vi "testRotGroupDOF.vi"(8 "error in (no error)":errorcluster) -> (0 "error out":errorcluster)   [LabVIEW 2016]
doc: "Test the rotation of degree of freedom (DOF) with the non-zero camera rotation angle."
uses:
  CamRot/CamRot.lvclass
  StrictDef/DofGroup.ctl
  <vilib>/addons/_JKI Toolkits/Caraya/classes/Test/Test.lvclass
  <vilib>/addons/_JKI Toolkits/Caraya/classes/Assert/Assert.lvclass
panel:
  in  "CamRot.lvclass":refnum<class "CamRot.lvclass">
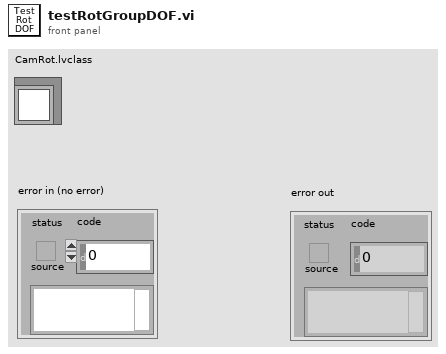
[diagram p1: front panel]
types:
  T1 = typedef "DofGroup.ctl" = enum16{"M2 Hex Pos", "Cam Hex Pos", "M1M3 Bend", "M2 Bend"}
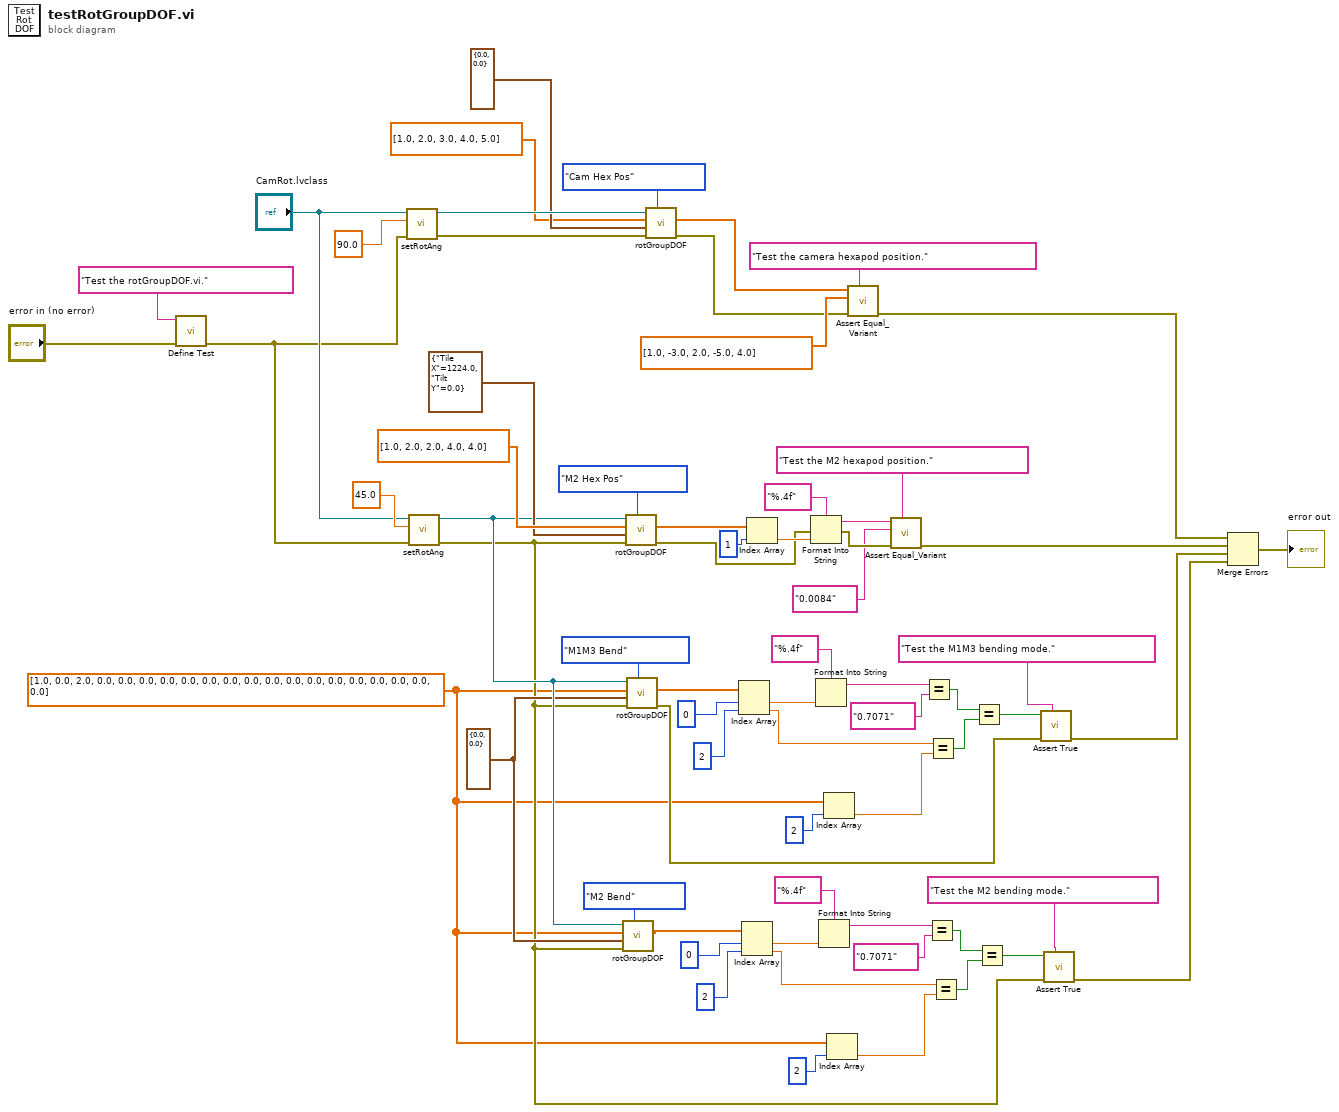
[diagram p0: block diagram]
diagram:
  w2 = dbl[] [1.0, 0.0, 2.0, 0.0, 0.0, 0.0, 0.0, 0.0, 0.0, 0.0, 0.0, 0.0, 0.0, 0.0, 0.0, 0.0, 0.0, 0.0, 0.0, 0.0] ("Hexapod DOF")
  w18 = cluster{"Tile X":dbl, "Tilt Y":dbl} {"Tile X"=0.0, "Tilt Y"=0.0} ("Tilt Angle (arcsec)")
  n1 = call <vilib>:"Define Test.vi"("error in (no error)"="error in (no error)", "Label (VI Title)"="Test the rotGroupDOF.vi.") -> ("error out"=w61:errorcluster)  [unwired: 9 in]
  n2 = call "setRotAng.vi"("error in (no error)"=w61, "Rotation Angle in Deg"=90.0, "CamRot in"="CamRot.lvclass") -> ("error out"=w45:errorcluster, "CamRot out"=w49:refnum<class "CamRot.lvclass">)  [unwired: 7 in]
  n3 = call "setRotAng.vi"("error in (no error)"=w61, "Rotation Angle in Deg"=45.0, "CamRot in"="CamRot.lvclass") -> ("error out"=w3:errorcluster, "CamRot out"=w19:refnum<class "CamRot.lvclass">)  [unwired: 7 in]
  n4 = call "rotGroupDOF.vi"("DOF Group"=DofGroup."M2 Bend", "error in (no error)"=w3, "Tilt Angle (arcsec)"=w18, "State in DOF"=w2, "CamRot in"=w19) -> ("Rotated State in DOF"=w4:dbl[])  [unwired: 4 in, 2 out]
  n5 = call "rotGroupDOF.vi"("DOF Group"=DofGroup."M2 Hex Pos", "error in (no error)"=w3, "Tilt Angle (arcsec)"=cluster{"Tile X":dbl, "Tilt Y":dbl} {"Tile X"=1224.0, "Tilt Y"=0.0}, "State in DOF"=dbl[] [1.0, 2.0, 2.0, 4.0, 4.0] ("Hexapod DOF"), "CamRot in"=w19) -> ("error out"=w39:errorcluster, "Rotated State in DOF"=w38:dbl[])  [unwired: 4 in, 1 out]
  n6 = call "rotGroupDOF.vi"("DOF Group"=DofGroup."M1M3 Bend", "error in (no error)"=w3, "Tilt Angle (arcsec)"=w18, "State in DOF"=w2, "CamRot in"=w19) -> ("error out"=w23:errorcluster, "Rotated State in DOF"=w36:dbl[])  [unwired: 4 in, 1 out]
  n7 = call "rotGroupDOF.vi"("DOF Group"=DofGroup."Cam Hex Pos", "error in (no error)"=w45, "Tilt Angle (arcsec)"=cluster{"Tile X":dbl, "Tilt Y":dbl} {"Tile X"=0.0, "Tilt Y"=0.0}, "State in DOF"=dbl[] [1.0, 2.0, 3.0, 4.0, 5.0] ("Hexapod DOF"), "CamRot in"=w49) -> ("error out"=w43:errorcluster, "Rotated State in DOF"=w44:dbl[])  [unwired: 4 in, 1 out]
  n8 = Index Array(array=w36, index #1=0 ("index"), index #2=2 ("index")) -> (element #1=w32:dbl, element #2=w29:dbl)
  n9 = Index Array(array=w4, index #1=0 ("index"), index #2=2 ("index")) -> (element #1=w14:dbl, element #2=w11:dbl)
  n10 = Index Array(array=w38, index=1) -> (element=w56:dbl)
  n11 = Format Into String(format string="%.4f" ("initial string"), error in=w39, w56) -> (resulting string=w54:string, error out=w52:errorcluster)  [unwired: 1 in]
  n12 = Format Into String(format string="%.4f" ("initial string"), w32) -> (resulting string=w31:string)  [unwired: 2 in, 1 out]
  n13 = Format Into String(format string="%.4f" ("initial string"), w14) -> (resulting string=w13:string)  [unwired: 2 in, 1 out]
  n14 = Index Array(array=w2, index=2) -> (element=w27:dbl)
  n15 = Index Array(array=w2, index=2) -> (element=w9:dbl)
  n16 = call <vilib>:"Assert Equal_Variant.vi"("Label"="Test the camera hexapod position.", "error in (no error)"=w43, "Y"=dbl[] [1.0, -3.0, 2.0, -5.0, 4.0] ("Hexapod DOF"), "X"=w44) -> ("error out"=w58:errorcluster)  [unwired: 7 in]
  n17 = call <vilib>:"Assert Equal_Variant.vi"("Label"="Test the M2 hexapod position.", "error in (no error)"=w52, "Y"="0.0084" ("Label"), "X"=w54) -> ("error out"=w51:errorcluster)  [unwired: 7 in]
  n18 = Equal?(x=w31, y="0.7071") -> (x = y?=w26:bool)
  n19 = Equal?(x=w13, y="0.7071") -> (x = y?=w8:bool)
  n20 = Equal?(x=w29, y=w27) -> (x = y?=w25:bool)
  n21 = Equal?(x=w11, y=w9) -> (x = y?=w7:bool)
  n22 = Equal?(x=w26, y=w25) -> (x = y?=w24:bool)
  n23 = Equal?(x=w8, y=w7) -> (x = y?=w6:bool)
  n24 = call <vilib>:"Assert True.vi"("Label"="Test the M1M3 bending mode.", "error in (no error)"=w23, "True?"=w24) -> ("error out"=w21:errorcluster)  [unwired: 8 in]
  n25 = call <vilib>:"Assert True.vi"("Label"="Test the M2 bending mode.", "error in (no error)"=w3, "True?"=w6) -> ("error out"=w1:errorcluster)  [unwired: 8 in]
  n26 = Merge Errors(w58, w51, w21, w1) -> (→"error out":errorcluster)
